vi "Update Paramater Value and Time.vi"(8 "error in (no error)":errorcluster, 9 "Value":dbl format="%#_13g", 10 "Start t":refnum<vi>, 11 "Current Sweep Value":refnum<vi>) -> (0 "error out":errorcluster)   [LabVIEW 2024]
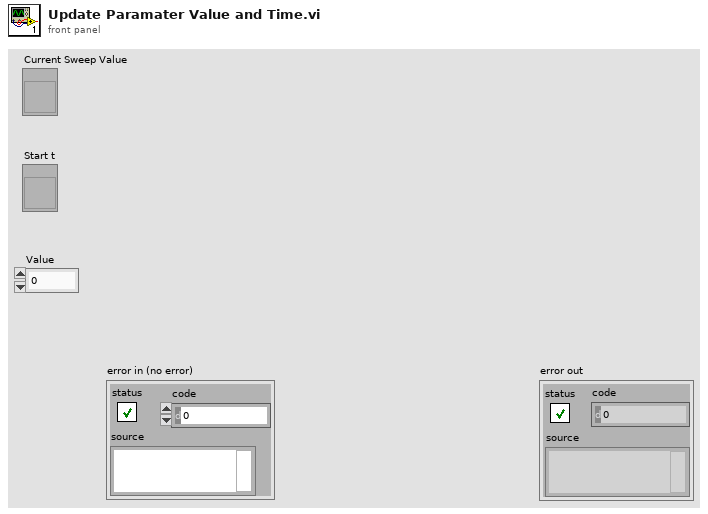
[diagram p1: front panel]
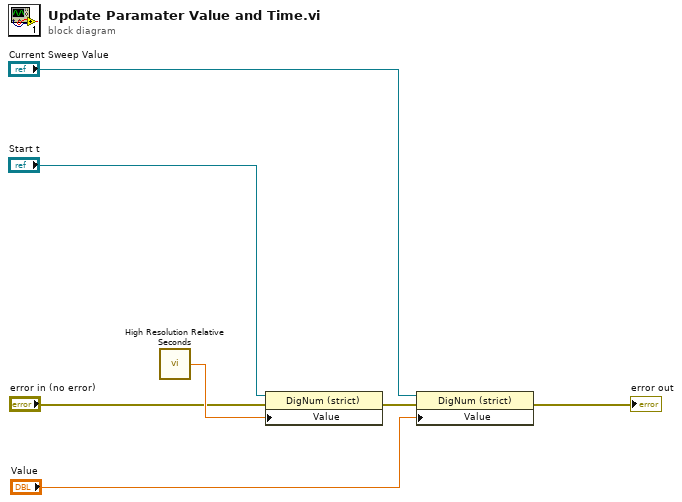
[diagram p0: block diagram]
diagram:
  n1 = call <vilib>:"High Resolution Relative Seconds.vi"() -> ("relative seconds"=w6:dbl)
  n2 = property class="DigNum (strict)"(reference="Start t", error in="error in (no error)", "Value"=w6) -> (error out=w7:errorcluster)  [unwired: 1 out]
  n3 = property class="DigNum (strict)"(reference="Current Sweep Value", error in=w7, "Value"="Value") -> (error out=→"error out":errorcluster)  [unwired: 1 out]
